vi "Run.vi"(7 "Team Index":i32, 8 "Column":i32, 9 "Row":i32, 10 "View":i32[](array[numeric]) caption="View (Team Index, -1: empty)", 11 "Trek In":refnum<class "Trek.lvclass">) -> (0 "Replicated":refnum<class "Square.lvclass">, 1 "Direction":T1, 2 "Action":T2, 3 "Trek Out":refnum<class "Square.lvclass">)   [LabVIEW 2016, in "Trek.lvclass"]
uses:
  Trek.lvclass
  C:/Users/Events/Desktop/SquareBattle/Square/Square.lvclass
  Square/Square.lvclass
  Type Defs/Action Enum.ctl
  Type Defs/Direction Enum.ctl
  Trek.lvclass/Trek.ctl
  Common/Position.ctl
  SubVIs/Read-Only Globals.vi
  SubVIs/Globals (private).vi
  Common/Common.lvlib
  Type Defs/SB Type Defs.lvlib
panel:
  # "NW\nN\nNE\nE\nSE\nS\nSW\nW"
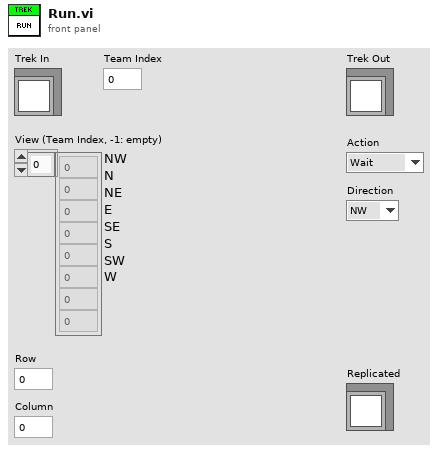
[diagram p1: front panel]
types:
  T1 = typedef "SB Type Defs.lvlib/Direction Enum.ctl" = enum16{"NW", "N", "NE", "E", "SE", "S", "SW", "W"}
  T2 = typedef "SB Type Defs.lvlib/Action Enum.ctl" = enum16{"Wait", "Move", "Attack", "Replicate"}
  T3 = typedef "Common.lvlib/Map DVR.ctl" = refnum<data-value>
  T4 = typedef "Common.lvlib/Position.ctl" = cluster{"Column":i32, "Row":i32}
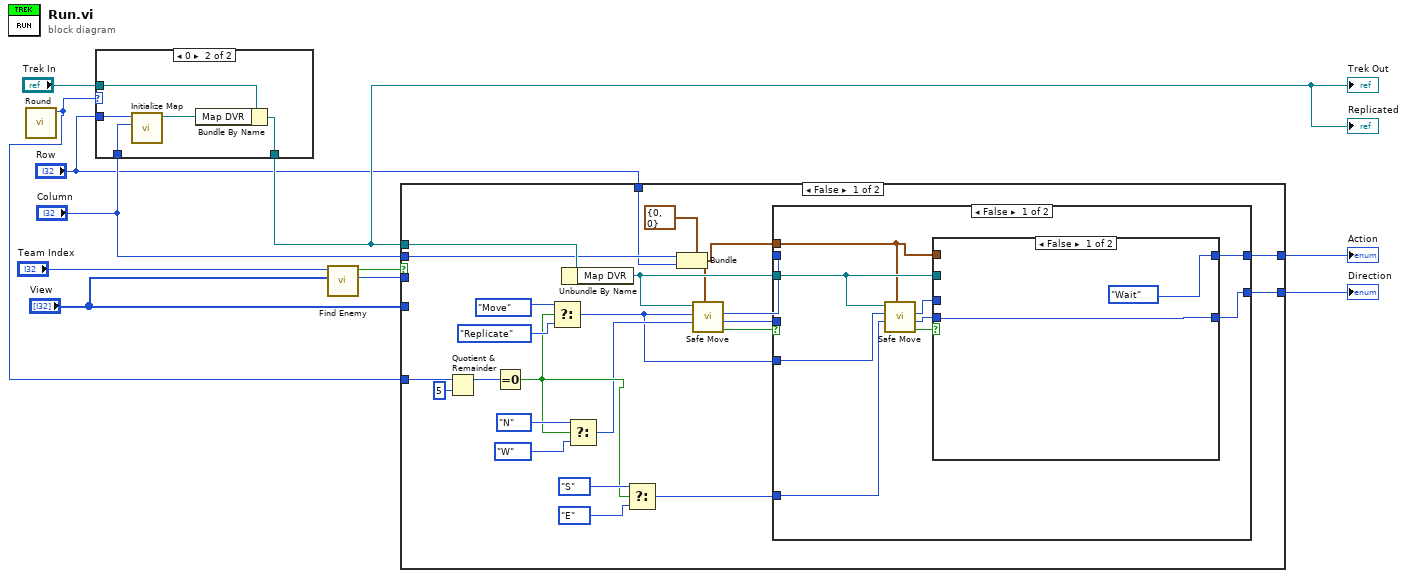
[diagram p0: block diagram]
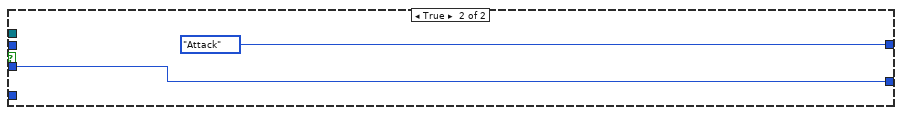
[diagram p5: hidden frame]
diagram:
  n1 = call "Round.vi"() -> ("Round"=w1:i32)  [unwired: 11 in]
  n2 = case shown="0" w1 {
    tunnel: "Trek In" -> [w12 w17]
    tunnel: "Row" -> [_ w15]
    tunnel: "Column" -> [_ w14]
    tunnel: [w12 w13] -> w4
    frame Default {
    }
    frame 0 {
      n3 = call "Initialize Map.vi"("Column"=w14, "Row"=w15) -> ("Map DVR"=w16:T3)  [unwired: 9 in]
      n4 = Bundle By Name(cluster=w17, "Map DVR"=w16) -> (w13:refnum<class "Trek.lvclass">)
    }
  }
  "Trek Out" <- w4
  "Replicated" <- w4
  n5 = call "Find Enemy.vi"("View"="View", "Team Index"="Team Index") -> ("Direction"=w9:T1, "Found Enemy?"=w10:bool)  [unwired: 7 in, 1 out]
  n6 = case shown="False" w10 {
    tunnel: w9 -> [_ w57]
    tunnel: [w37 Action_Enum."Attack" ("Action")] -> w8
    tunnel: [w38 w57] -> w7
    tunnel: "View" -> [_ _]
    tunnel: w4 -> [w41 _]
    tunnel: "Column" -> [w34 _]
    tunnel: "Row" -> [w33 _]
    tunnel: w1 -> [w32 _]
    frame False {
      n7 = Quotient & Remainder(x=w32, y=5) -> (x-y*floor(x/y)=w30:i32)  [unwired: 1 out]
      n8 = Equal To 0?(x=w30) -> (x = 0?=w21:bool)
      n9 = Select(t=Action_Enum."Move" ("Desired Action"), s=w21, f=Action_Enum."Replicate" ("Desired Action")) -> (s? t:f=w18:T2)
      n10 = Unbundle By Name(w41) -> ("Map DVR"=w25:T3)
      n11 = Select(t=Direction_Enum."N" ("Direction in"), s=w21, f=Direction_Enum."W" ("Direction in")) -> (s? t:f=w19:T1)
      n12 = Select(t=Direction_Enum."S" ("Direction in"), s=w21, f=Direction_Enum."E" ("Direction in")) -> (s? t:f=w20:T1)
      n13 = Bundle(cluster=T4 {"Column"=0, "Row"=0} ("Position in"), "Column"=w34, "Row"=w33) -> (w24:T4)
      n14 = call "Safe Move.vi"("Position in"=w24, "Direction in"=w19, "Desired Action"=w18, "Map DVR"=w25) -> ("Accepted?"=w40:bool, "Direction"=w39:T1, "Action"=w36:T2)  [unwired: 4 in, 1 out]
      n15 = case shown="False" w40 {
        tunnel: w39 -> [_ w56]
        tunnel: [w49 w56] -> w38
        tunnel: [w47 w55] -> w37
        tunnel: w36 -> [_ w55]
        tunnel: w25 -> [w45 _]
        tunnel: w24 -> [w44 _]
        tunnel: w20 -> [w43 _]
        tunnel: w18 -> [w42 _]
        frame False {
          n16 = call "Safe Move.vi"("Position in"=w44, "Direction in"=w43, "Desired Action"=w42, "Map DVR"=w45) -> ("Accepted?"=w50:bool, "Direction"=w48:T1, "Action"=w46:T2)  [unwired: 4 in, 1 out]
          n17 = case shown="False" w50 {
            tunnel: [w51 w54] -> w49
            tunnel: w48 -> [w51 w54]
            tunnel: [Action_Enum."Wait" ("Action") w53] -> w47
            tunnel: w46 -> [_ w53]
            tunnel: w45 -> [_ _]
            tunnel: w44 -> [_ _]
            frame False {
            }
            frame True {
            }
          }
        }
        frame True {
        }
      }
    }
    frame True {
    }
  }
  "Action" <- w8
  "Direction" <- w7
